vi "KG number of mfc.vi"(8 "Fehler (Eingang, kein Fehler)":errorcluster, 11 "VISA-Ressourcenname":refnum<visa-resource-name>) -> (0 "Fehler (Ausgang)":errorcluster, 1 "Kommando gesendet":string, 2 "number of mfc":dbl, 3 "VISA-Ressourcenname (Ausgang)":refnum<visa-resource-name>)   [LabVIEW 2020, in "Linearisierung v2.lvlib" / "Gasteiler.lvlib" / "HovaCAL_Interface.lvlib" / "KGN.lvlib" / "get.lvlib"]
uses:
  get.lvlib
  KGN.lvlib
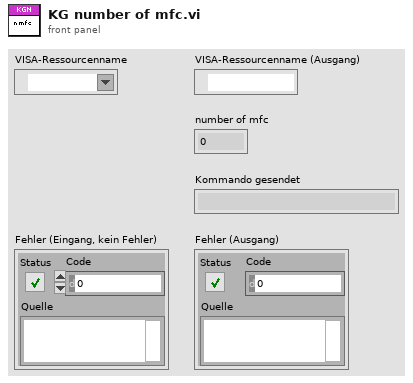
[diagram p1: front panel]
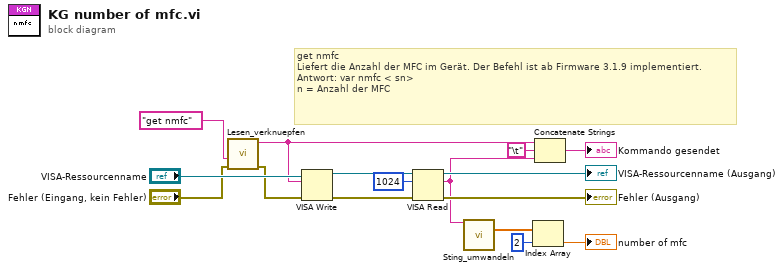
[diagram p0: block diagram]
diagram:
  # "get nmfc\nLiefert die Anzahl der MFC im Gerät. Der Befehl ist ab Firmware 3.1.9 implementiert.\nAntwort: var nmfc < sn>\nn = Anzahl der MFC"
  n1 = call "Lesen_verknuepfen.vi"("error in (no error)"="Fehler (Eingang, kein Fehler)", "Order"="get nmfc" ("Schreibpuffer")) -> ("error out"=w9:errorcluster, "Verknüpfter String"=w3:string)  [unwired: 8 in]
  n2 = VISA Write(VISA resource name="VISA-Ressourcenname", write buffer=w3, error in (no error)=w9) -> (VISA resource name out=w16:refnum<visa-resource-name>, error out=w15:errorcluster)  [unwired: 1 out]
  n3 = VISA Read(VISA resource name=w16, byte count=u32 1024 ("Byte-Anzahl"), error in (no error)=w15) -> (VISA resource name out=→"VISA-Ressourcenname (Ausgang)":refnum<visa-resource-name>, read buffer=w1:string, error out=→"Fehler (Ausgang)":errorcluster)  [unwired: 1 out]
  n4 = call "Sting_umwandeln.vi"("Lesepuffer"=w1) -> ("Zahl array"=w6:dbl[])  [unwired: 8 in, 6 out]
  n5 = Index Array(array=w6, index=2 ("Index")) -> (element=→"number of mfc":dbl)
  n6 = Concatenate Strings(w3, "\t", w1) -> (→"Kommando gesendet":string)
